vi "getSelected.vi"(10 "Weight":i32[](array[numeric]), 11 "Predict":i32[](array[numeric])) -> (3 "selected":i32)   [LabVIEW 2014]
panel:
  out "subarray":i32[](array[numeric])
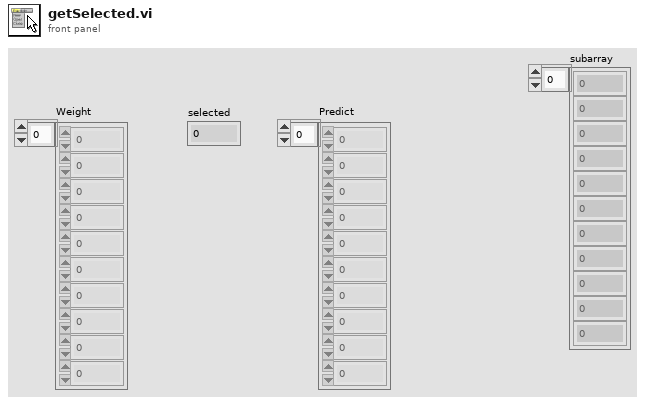
[diagram p1: front panel]
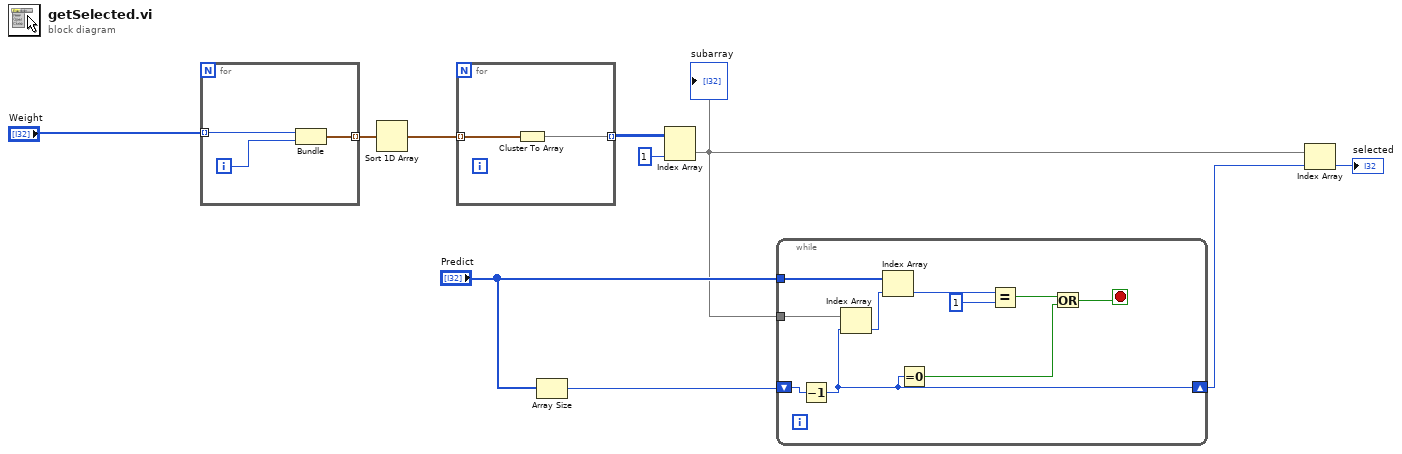
[diagram p0: block diagram]
diagram:
  n1 = for {
    tunnel: "Weight" -> [w13] mode=indexing
    tunnel: [w12] -> w10 mode=indexing
    i -> [w11]
    n2 = Bundle("Numeric"=w13, w11) -> (w12:cluster{"Numeric":i32, i32})  [unwired: 1 in]
  }
  n3 = Sort 1D Array(array=w10) -> (sorted array=w9:cluster{"Numeric":i32, i32}[])
  n4 = for {
    tunnel: w9 -> [w15] mode=indexing
    tunnel: [w14] -> w8 mode=indexing
    n5 = Cluster To Array(cluster=w15) -> (array=w14:i32[])
  }
  n6 = Array Size(array="Predict") -> (size(s)=w3:i32)
  n7 = Index Array(array=w8, index (col)=1 ("index")) -> (element=w2:i32[])  [unwired: 1 in]
  "subarray" <- w2
  n8 = while {
    tunnel: "Predict" -> [w19]
    shift-right: [w21] -> w1
    shift-left: w3 -> [w23]
    tunnel: w2 -> [w20]
    stop <- w25 stop-if-true
    n9 = Decrement(x=w23) -> (x-1=w21:i32)
    n10 = Index Array(array=w20, index=w21) -> (element=w18:i32)
    n11 = Index Array(array=w19, index=w18) -> (element=w17:i32)
    n12 = Equal To 0?(x=w21) -> (x = 0?=w22:bool)
    n13 = Equal?(x=w17, y=1) -> (x = y?=w24:bool)
    n14 = Or(x=w24, y=w22) -> (x .or. y?=w25:bool)
  }
  n15 = Index Array(array=w2, index=w1) -> (element=→"selected":i32)
